vi "Insert Data.vi"(7 "Group":string, 8 "error in":errorcluster, 9 "Data":variant, 10 "tag":string, 11 "CVT Session In":T1) -> (0 "error out":errorcluster, 3 "CVT Session Out":T1)   [LabVIEW 2015, in "CVT.lvclass"]
uses:
  CVT.lvclass
  <userlib>/_Session Fwk/Typedefs/Session Handle.ctl
  <userlib>/_Session Fwk/Session - Root.lvclass
  CVT.lvclass/CVT.ctl
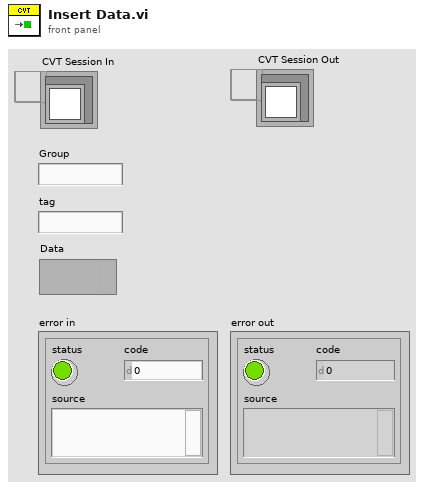
[diagram p1: front panel]
types:
  T1 = typedef "Session - Root.lvclass/Session Handle.ctl" = refnum<data-value>
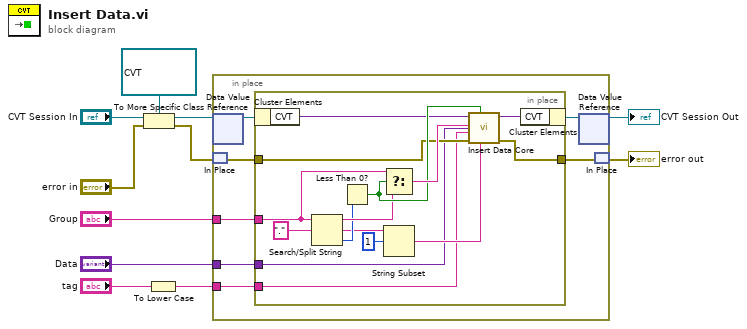
[diagram p0: block diagram]
diagram:
  n1 = To More Specific Class(target class=refnum<data-value> refnum ("CVT Session In"), reference="CVT Session In", error in="error in") -> (specific class reference=w9:refnum<data-value>, error out=w7:errorcluster)
  n2 = To Lower Case(string="tag") -> (all lower case string=w1:string)
  n3 = in-place {
    in-place-border: "Group" -> [w18]
    in-place-border: w1 -> [w17]
    in-place-border: "Data" -> [w16]
    n4 = in-place-dvr #1(w9) -> (w15:refnum<class "CVT.lvclass">)  [unwired: 1 out]
    n5 = in-place-match #2(w7) -> (w14:errorcluster)
    n6 = in-place {
      in-place-border: w18 -> [w20]
      in-place-border: w17 -> [w19]
      in-place-border: w16 -> [w21]
      in-place-border: w14 -> [w22]
      in-place-border: [w23] -> w12
      n7 = in-place-cluster #3(w15) -> ("CVT"=w25:variant)
      n8 = Search/Split String(string=w20, search string/char (-)="." ("regular expression")) -> (substring before match=w31:string, match + rest of string=w28:string, offset of match=w30:i32)  [unwired: 1 in]
      n9 = Less Than 0?(x=w30) -> (x < 0?=w32:bool)
      n10 = Select(t=w20, s=w32, f=w31) -> (s? t:f=w33:string)
      n11 = String Subset(string=w28, offset (0)=1) -> (substring=w26:string)  [unwired: 1 in]
      n12 = call "Insert Data Core.vi"("Data"=w21, "Nested Group"=w26, "Nested?"=w32, "error in"=w22, "tag"=w19, "Group"=w33, "CVT In"=w25) -> ("error out"=w23:errorcluster, "CVT Out"=w24:variant)  [unwired: 2 in]
      n13 = in-place-cluster #3("CVT"=w24) -> (w13:refnum<class "CVT.lvclass">)
    }
    n14 = in-place-dvr #1(w13) -> (→"CVT Session Out":refnum<data-value>)  [unwired: 1 out]
    n15 = in-place-match #2(w12) -> (→"error out":errorcluster)
  }
